vi "Save Events to DB.vi"(0 "Array":string[][](array[string]), 1 "db file":path=path "D:/SQL Database/Gtron Database.db", 3 "error in":errorcluster) -> (10 "error out":errorcluster)   [LabVIEW 2019, in "DataLogger.lvclass"]
doc: "Save Events details"
uses:
  DataLogger.lvclass
  <vilib>/drjdpowell/SQLite Library/SQL Statement/SQL Statement.lvclass
  <vilib>/drjdpowell/SQLite Library/SQL Connection/Connection.lvclass
  <vilib>/drjdpowell/SQLite Library/SQL Connection/Open (path).vi
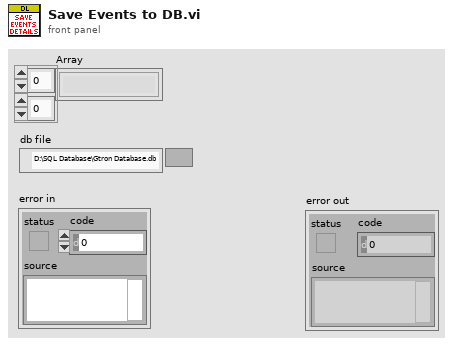
[diagram p1: front panel]
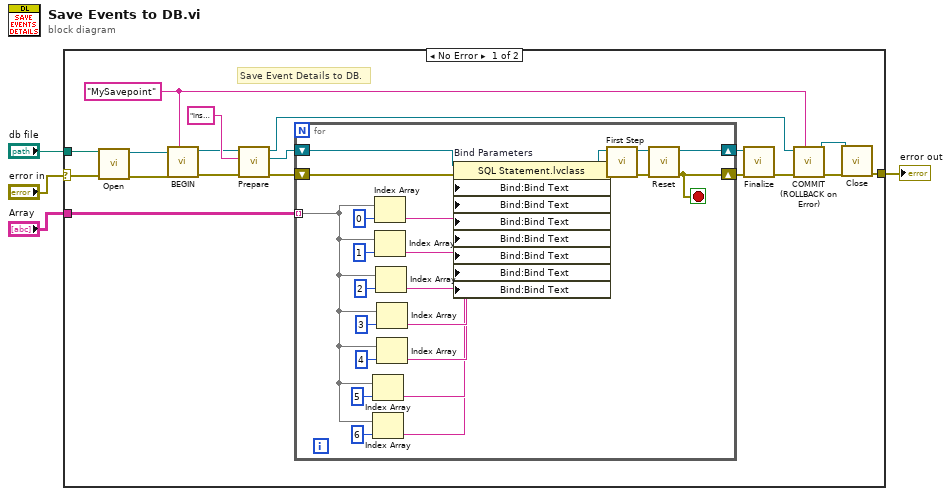
[diagram p0: block diagram]
diagram:
  n1 = case shown="No Error" "error in" {
    selector: "error in" -> [w7 w46]
    tunnel: "db file" -> [w6 _]
    tunnel: [w10 w46] -> w4
    tunnel: "Array" -> [w5 _]
    frame No Error {
      w15 = "MySavepoint" ("Savepoint name")
      # "Save Event Details to DB."
      n2 = call-poly <vilib>:"Open.vi"("error in (no error)"=w7, "db file"=w6) -> ("error out"=w8:errorcluster, "SQLite Connection"=w9:refnum<class "Connection.lvclass">)  [unwired: 8 in]
      n3 = call <vilib>:"BEGIN.vi"("Savepoint name"=w15, "error in (no error)"=w8, "Connection in"=w9) -> ("error out"=w16:errorcluster, "Connection out"=w17:refnum<class "Connection.lvclass">)  [unwired: 7 in]
      n4 = call <vilib>:"Prepare.vi"("error in (no error)"=w16, "SQL"="insert into EventDetails  VALUES (?,?,?,?,?,?,?)" ("INSERT statement"), "SQLite Connection in"=w17) -> ("error out"=w21:errorcluster, "SQL Statement"=w22:refnum<class "SQL Statement.lvclass">, "SQLite Connection"=w14:refnum<class "Connection.lvclass">)  [unwired: 4 in, 2 out]
      n5 = for "For each set of parameters to be inserted..." {
        shift-right: [w43] -> w19
        shift-left: w22 -> [w45]
        shift-right: [w42] -> w18
        shift-left: w21 -> [w44]
        tunnel: w5 -> [w41] mode=indexing
        stop <- w42 stop-if-true
        n6 = Index Array(array=w41, index=5) -> (element=w24:string)
        n7 = Index Array(array=w41, index=6) -> (element=w23:string)
        n8 = Index Array(array=w41, index=0) -> (element=w29:string)
        n9 = Index Array(array=w41, index=1) -> (element=w28:string)
        n10 = Index Array(array=w41, index=2) -> (element=w27:string)
        n11 = Index Array(array=w41, index=3) -> (element=w26:string)
        n12 = Index Array(array=w41, index=4) -> (element=w25:string)
        n13 = property on="Bind Parameters" class="SQL Statement.lvclass"(reference=w45, error in=w44, "Bind:Bind Text"=w29, "Bind:Bind Text"=w28, "Bind:Bind Text"=w27, "Bind:Bind Text"=w26, "Bind:Bind Text"=w25, "Bind:Bind Text"=w24, "Bind:Bind Text"=w23) -> (reference out=w40:refnum<class "SQL Statement.lvclass">, error out=w39:errorcluster)
        n14 = call <vilib>:"First Step.vi"("error in (no error)"=w39, "SQL Statement in"=w40) -> ("error out"=w38:errorcluster, "SQL Statement"=w37:refnum<class "SQL Statement.lvclass">)  [unwired: 7 in, 1 out]
        n15 = call <vilib>:"Reset.vi"("error in (no error)"=w38, "SQL Statement in"=w37) -> ("error out"=w42:errorcluster, "SQL Statement"=w43:refnum<class "SQL Statement.lvclass">)  [unwired: 8 in]
      }
      n16 = call <vilib>:"Finalize.vi"("error in (no error)"=w18, "SQL Statement in"=w19) -> ("error out"=w13:errorcluster)  [unwired: 9 in]
      n17 = call <vilib>:"COMMIT (ROLLBACK on Error).vi"("Savepoint name"=w15, "error in (no error)"=w13, "Connection in"=w14) -> ("error out"=w12:errorcluster, "Connection out"=w11:refnum<class "Connection.lvclass">)  [unwired: 7 in]
      n18 = call-dynamic "Close.vi"("error in (no error)"=w12, "SQLite Connection in"=w11) -> ("error out"=w10:errorcluster)  [unwired: 9 in]
    }
    frame Error {
    }
  }
  "error out" <- w4
